vi "Day10-03_OCR.vi"() -> ()   [LabVIEW 2021]
uses:
  <vilib>/vision/NI_Vision_Development_Module.lvlib
panel:
  in  "정지":bool
  out "Character Value2":string
  in  "Character Index":dbl
  out "Read String":string
  in  "학습 파일 확인":bool
  in  "Character Value":string
  in  "저장":bool
  in  "File Path":path
  in  "학습":bool
  in  "판별":bool
  out "Image":T1(plugin-control)
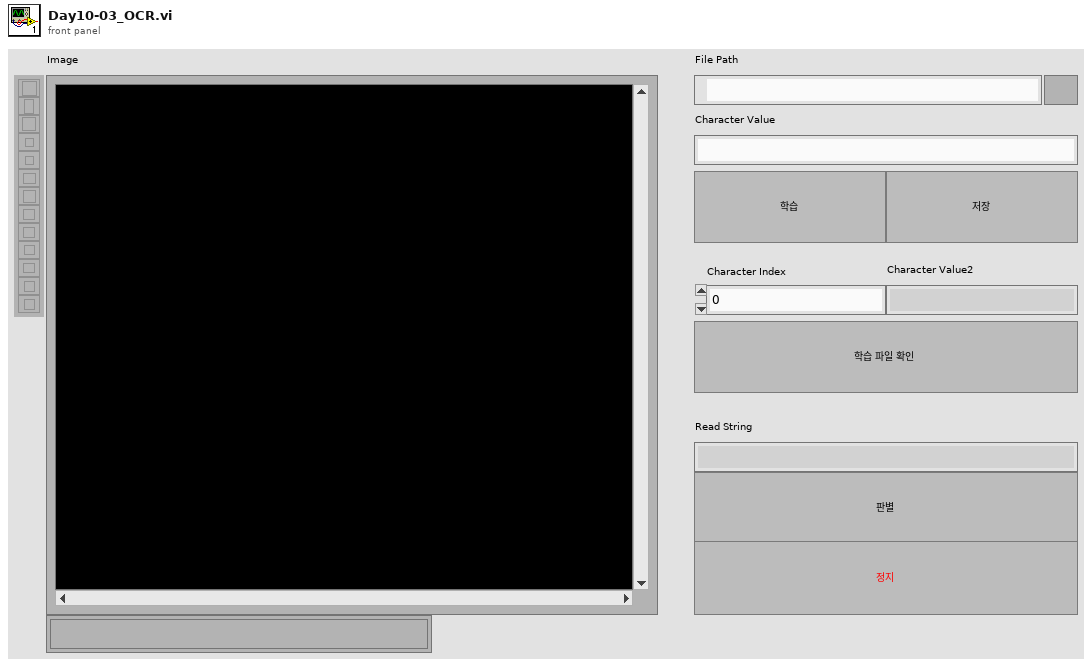
[diagram p1: front panel]
types:
  T1 = typedef "IMAQ Image.ctl" = refnum<image>
  T2 = typedef "ROI Descriptor" = cluster{"Global Rectangle":i32[], "Contours":cluster{"ID":enum32{"External", "Internal"}, "Type":u32, "Coordinates":i32[]}[]}
  T3 = cluster{"학습파일":path, "샘플 파일":path, "ROI Descriptor Out":T2}
  T4 = typedef "Image Type" = u32
  T5 = typedef "IMAQ OCR Session.ctl" = refnum<k1>
  T6 = cluster{"Global Rectangle":i32[], "Contours":cluster{"ID":enum32{"External", "Internal"}, "Type":u32, "Coordinates":i32[]}[]}
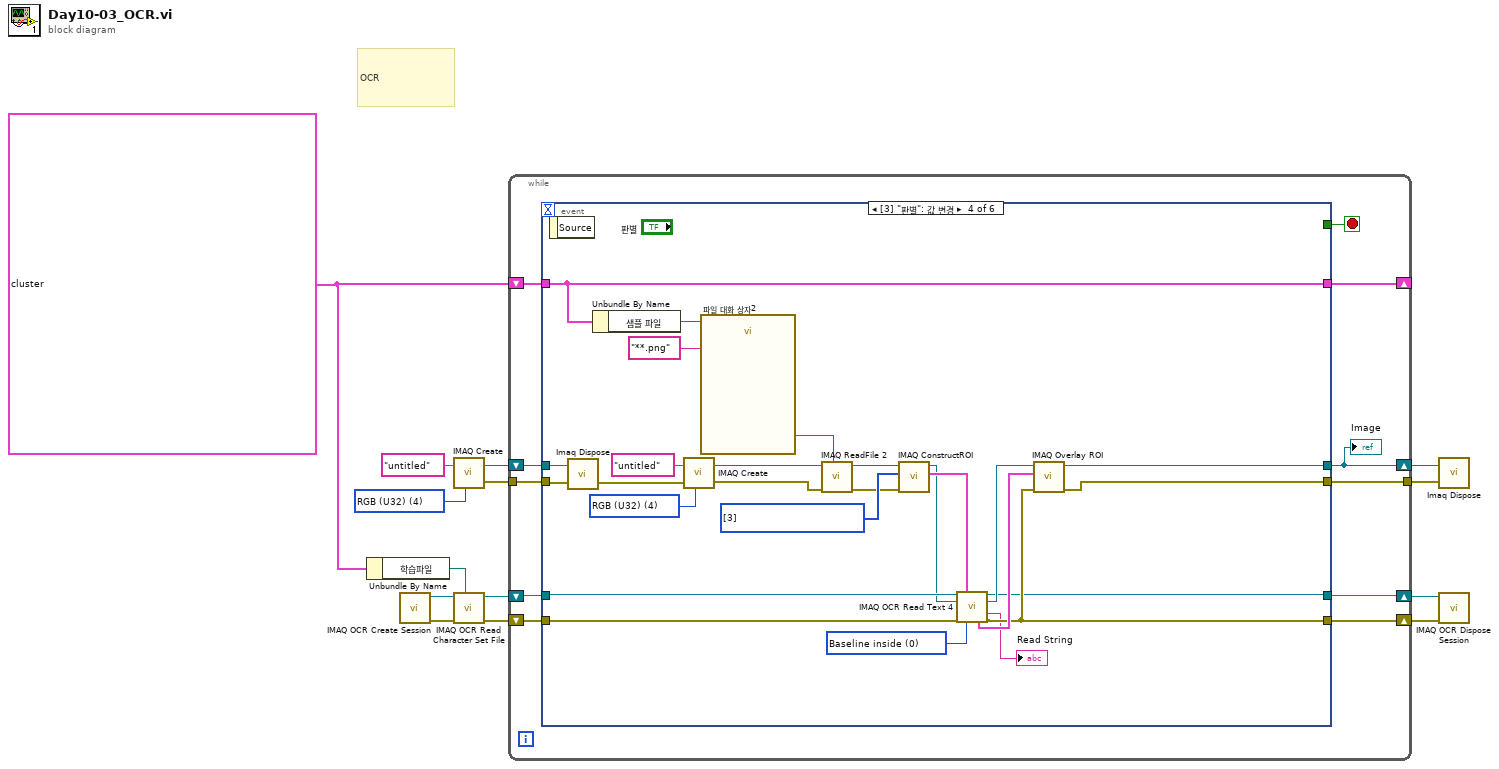
[diagram p0: block diagram]
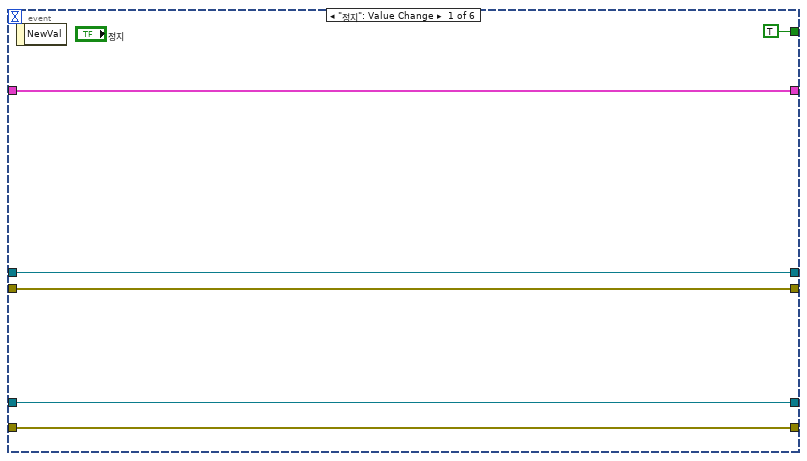
[diagram p2: hidden frame]
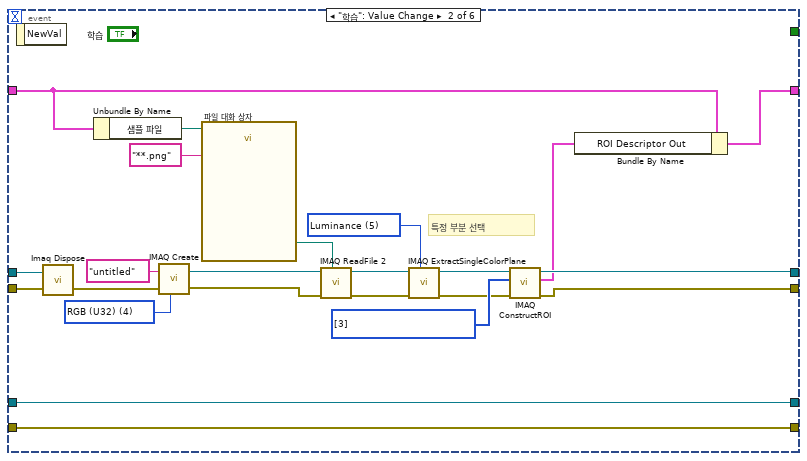
[diagram p3: hidden frame]
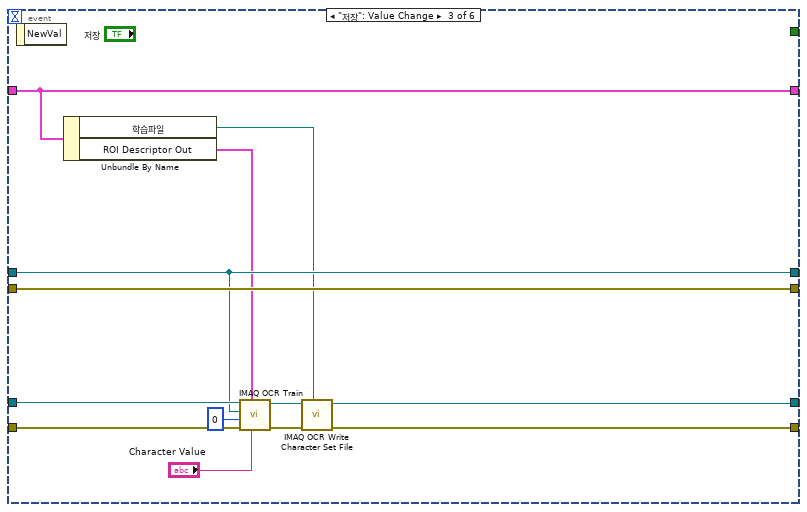
[diagram p4: hidden frame]
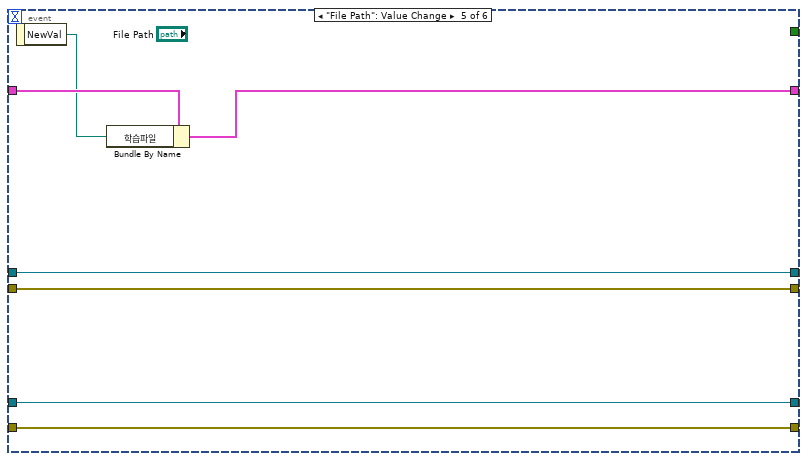
[diagram p5: hidden frame]
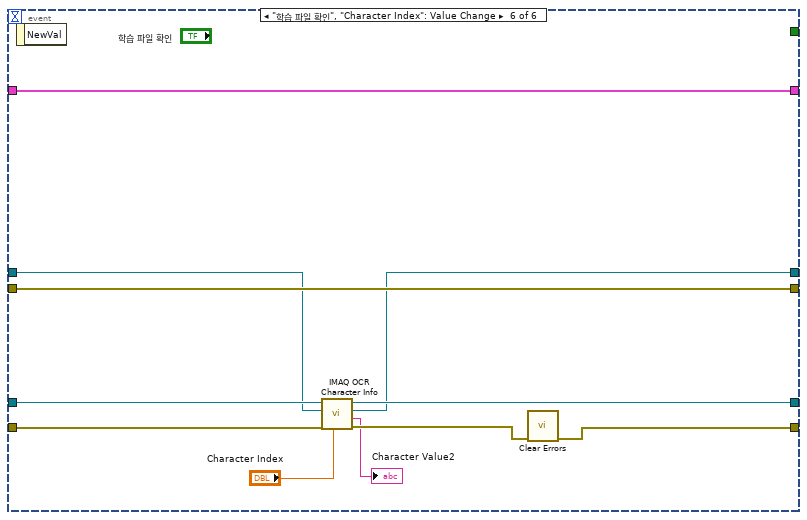
[diagram p6: hidden frame]
diagram:
  w6 = T3 {"학습파일"=path "C:/Embedded_System/04_LabVIEW/Programming_SourceCode/LabVIEW/이미지파일/OCR/학습.abc", "샘플 파일"=path "C:/Embedded_System/04_LabVIEW/Programming_SourceCode/LabVIEW/이미지파일/OCR", "ROI Descriptor Out"={"Global Rectangle"=[], "Contours"=[]}}
  w12 = T4 4 items=["Grayscale (U8)", "Grayscale (I16)", "Grayscale (SGL)", "Complex (CSG)", "RGB (U32)", "HSL (U32)", "RGB (U64)", "Grayscale (U16)"] ("Image Type")
  # "OCR"
  n1 = Unbundle By Name(w6) -> ("학습파일"=w4:path)
  n2 = call "IMAQ OCR Create Session"() -> ("error out"=w7:errorcluster, "IMAQ OCR Session"=w8:T5)  [unwired: 10 in]
  n3 = call "IMAQ Create"("Image Name"="untitled", "Image Type"=w12) -> ("New Image"=w14:T1, "error out"=w13:errorcluster)  [unwired: 2 in, 1 out]
  n4 = call "IMAQ OCR Read Character Set File"("File Path"=w4, "error in (no error)"=w7, "IMAQ OCR Session"=w8) -> ("error out"=w5:errorcluster, "IMAQ OCR Session (dup)"=w9:T5)  [unwired: 6 in, 1 out]
  n5 = while {
    shift-right: [w22] -> _
    shift-left: w6 -> [w23]
    shift-right: [w19] -> w10
    shift-left: w14 -> [w24]
    shift-right: [w18] -> w2
    shift-left: w9 -> [w21]
    tunnel: w13 -> [w25]
    shift-right: [w16] -> w1
    shift-left: w5 -> [w17]
    tunnel: [w15] -> w3
    stop <- w20 stop-if-true
    n6 = event shown="[3] \"판별\": 값 변경" {
      selector: _ -> [_ _ _ _ _ _]
      dyn-events: _ -> [_ _ _ _ _ _]
      timeout: _ -> [_ _ _ _ _ _]
      tunnel: w25 -> [w26 w47 w67 w83 w95 w111]
      tunnel: w24 -> [w31 w48 w57 w84 w97 w102]
      tunnel: [w31 w39 w57 w79 w97 w101] -> w19
      tunnel: w23 -> [w30 w52 w66 w91 w100 w110]
      tunnel: [w30 w51 w66 w91 w98 w110] -> w22
      tunnel: [w29 w45 w63 w71 w96 w106] -> w18
      tunnel: w21 -> [w29 w45 w65 w74 w96 w109]
      tunnel: [TRUE _ _ _ _ _] -> w20
      tunnel: w17 -> [w27 w44 w60 w73 w94 w108]
      tunnel: [w27 w44 w62 w72 w94 w105] -> w16
      tunnel: [w26 w38 w67 w78 w95 w111] -> w15
      event "정지": Value Change {
        n7 = event-data() -> ()  [unwired: 1 in, 1 out]
      }
      event "학습": Value Change {
        w33 = 5 items=["Red", "Green", "Blue", "Hue", "Saturation", "Luminance", "Value", "Intensity"] ("Color Plane")
        w42 = T4 4 items=["Grayscale (U8)", "Grayscale (I16)", "Grayscale (SGL)", "Complex (CSG)", "RGB (U32)", "HSL (U32)", "RGB (U64)", "Grayscale (U16)"] ("Image Type")
        w53 = u32[] [3] items=["No Selection", "Point", "Line", "Rectangle", "Oval", "Polygon", "Freehand Region", "Annulus", "Zoom", "Pan", "Broken Line", "Freehand Line", "Rotated Rectangle"] ("Tools")
        # "특정 부분 선택"
        n8 = event-data() -> ()  [unwired: 1 in, 1 out]
        n9 = call "Imaq Dispose"("Image"=w48, "error in (no error)"=w47) -> ("error out"=w46:errorcluster)  [unwired: 4 in]
        n10 = Unbundle By Name(w52) -> ("샘플 파일"=w50:path)
        n11 = call "IMAQ Create"("Image Name"="untitled", "Image Type"=w42, "error in (no error)"=w46) -> ("New Image"=w41:T1, "error out"=w40:errorcluster)  [unwired: 1 in, 1 out]
        n12 = call "파일 대화 상자"("start path"=w50, "pattern (all files)"="**.png") -> ("selected path"=w54:path)  [unwired: 10 in, 3 out]
        n13 = call "IMAQ ReadFile 2"("File Path"=w54, "error in (no error)"=w40, "Image"=w41) -> ("error out"=w35:errorcluster, "Image Out"=w37:T1)  [unwired: 4 in, 3 out]
        n14 = call "IMAQ ExtractSingleColorPlane"("Color Plane"=w33, "error in (no error)"=w35, "Image Src"=w37) -> ("error out"=w34:errorcluster, "Image Dst Out"=w36:T1)  [unwired: 7 in]
        n15 = call "IMAQ ConstructROI"("error in (no error)"=w34, "Tools"=w53, "Image"=w36) -> ("error out"=w38:errorcluster, "ROI Descriptor Out"=w32:T2, "Image Out (duplicate)"=w39:T1)  [unwired: 5 in, 1 out]
        n16 = Bundle By Name(cluster=w52, "ROI Descriptor Out"=w32) -> (w51:T3)
      }
      event "저장": Value Change {
        n17 = event-data() -> ()  [unwired: 1 in, 1 out]
        n18 = Unbundle By Name(w66) -> ("학습파일"=w56:path, "ROI Descriptor Out"=w55:T2)
        n19 = call "IMAQ OCR Train"("Character Value"="Character Value", "ROI Descriptor"=w55, "error in (no error)"=w60, "Object Index"=0, "Image"=w57, "IMAQ OCR Session"=w65) -> ("error out"=w61:errorcluster, "IMAQ OCR Session (dup)"=w64:T5)  [unwired: 3 in, 1 out]
        n20 = call "IMAQ OCR Write Character Set File"("File Path"=w56, "error in (no error)"=w61, "IMAQ OCR Session"=w64) -> ("error out"=w62:errorcluster, "IMAQ OCR Session (dup)"=w63:T5)  [unwired: 7 in]
      }
      event "판별": Value Change {
        w69 = u32 0 items=["Baseline inside", "Baseline outside"] ("Orientation")
        w87 = T4 4 items=["Grayscale (U8)", "Grayscale (I16)", "Grayscale (SGL)", "Complex (CSG)", "RGB (U32)", "HSL (U32)", "RGB (U64)", "Grayscale (U16)"] ("Image Type")
        w90 = u32[] [3] items=["No Selection", "Point", "Line", "Rectangle", "Oval", "Polygon", "Freehand Region", "Annulus", "Zoom", "Pan", "Broken Line", "Freehand Line", "Rotated Rectangle"] ("Tools")
        n21 = event-data() -> ()  [unwired: 1 in, 1 out]
        n22 = call "Imaq Dispose"("Image"=w84, "error in (no error)"=w83) -> ("error out"=w89:errorcluster)  [unwired: 4 in]
        n23 = Unbundle By Name(w91) -> ("샘플 파일"=w93:path)
        n24 = call "IMAQ Create"("Image Name"="untitled", "Image Type"=w87, "error in (no error)"=w89) -> ("New Image"=w86:T1, "error out"=w85:errorcluster)  [unwired: 1 in, 1 out]
        n25 = call "파일 대화 상자2"("start path"=w93, "pattern (all files)"="**.png") -> ("selected path"=w82:path)  [unwired: 10 in, 3 out]
        n26 = call "IMAQ ReadFile 2"("File Path"=w82, "error in (no error)"=w85, "Image"=w86) -> ("error out"=w80:errorcluster, "Image Out"=w81:T1)  [unwired: 4 in, 3 out]
        n27 = call "IMAQ ConstructROI"("error in (no error)"=w80, "Tools"=w90, "Image"=w81) -> ("ROI Descriptor Out"=w77:T2, "Image Out (duplicate)"=w70:T1)  [unwired: 5 in, 2 out]
        n28 = call "IMAQ OCR Read Text 4"("IMAQ OCR Session"=w74, "ROI Descriptor"=w77, "Image"=w70, "error in (no error)"=w73, "Orientation"=w69) -> ("IMAQ OCR Session (dup)"=w71:T5, "Image (dup)"=w76:T1, "Read String"=→"Read String":string, "ROI Bounding Characters"=w75:T6, "error out"=w72:errorcluster)  [unwired: 4 in, 2 out]
        n29 = call "IMAQ Overlay ROI"("error in (no error)"=w72, "ROI Descriptor"=w75, "Image"=w76) -> ("error out"=w78:errorcluster, "Image Out"=w79:T1)  [unwired: 7 in]
      }
      event "File Path": Value Change {
        n30 = event-data() -> ("NewVal"=w99:path)  [unwired: 1 in]
        n31 = Bundle By Name(cluster=w100, "학습파일"=w99) -> (w98:T3)
      }
      event "학습 파일 확인", "Character Index": Value Change {
        n32 = event-data() -> ()  [unwired: 1 in, 1 out]
        n33 = call "IMAQ OCR Character Info"("Character Index"="Character Index", "error in (no error)"=w108, "Character Image"=w102, "IMAQ OCR Session"=w109) -> ("error out"=w107:errorcluster, "Character Value"=→"Character Value2":string, "Character Image (out)"=w101:T1, "IMAQ OCR Session (dup)"=w106:T5)  [unwired: 2 in, 2 out]
        n34 = call <vilib>:"Clear Errors.vi"("error in (no error)"=w107) -> ("error out"=w105:errorcluster)  [unwired: 5 in, 1 out]
      }
    }
    "Image" <- w19
  }
  n35 = call "Imaq Dispose"("Image"=w10, "error in (no error)"=w3) -> ()  [unwired: 4 in, 1 out]
  n36 = call "IMAQ OCR Dispose Session"("error in (no error)"=w1, "IMAQ OCR Session"=w2) -> ()  [unwired: 9 in, 1 out]
